vi "Парал-рег.vi"(0 "d 1":bool, 1 "d 2":bool, 2 "d 3":bool, 3 "d 4":bool, 4 "d 5":bool, 7 "Reset":bool, 9 "C":bool) -> (14 "Q 0":bool, 15 "Q 1":bool, 16 "Q 2":bool, 17 "Q 3":bool, 18 "Q 4":bool)   [LabVIEW 2012]
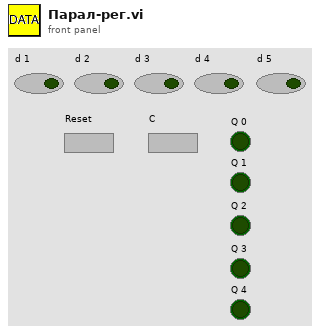
[diagram p1: front panel]
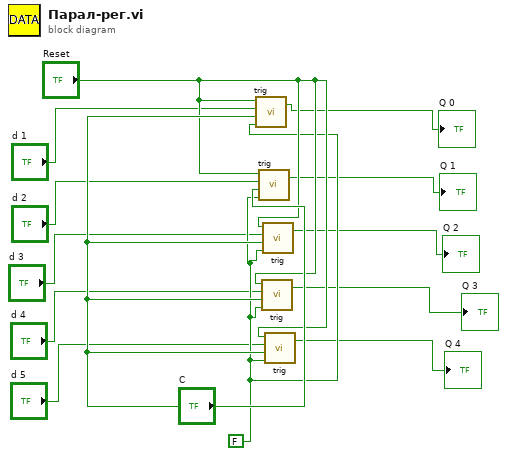
[diagram p0: block diagram]
diagram:
  w11 = FALSE
  n1 = call "trig.vi"("s"=w11, "c"="C", "d"="d 1", "r"="Reset") -> ("q"=→"Q 0":bool)  [unwired: 1 out]
  n2 = call "trig.vi"("s"=w11, "c"="C", "d"="d 2", "r"="Reset") -> ("q"=→"Q 1":bool)  [unwired: 1 out]
  n3 = call "trig.vi"("s"=w11, "c"="C", "d"="d 4", "r"="Reset") -> ("q"=→"Q 3":bool)  [unwired: 1 out]
  n4 = call "trig.vi"("s"=w11, "c"="C", "d"="d 3", "r"="Reset") -> ("q"=→"Q 2":bool)  [unwired: 1 out]
  n5 = call "trig.vi"("s"=w11, "c"="C", "d"="d 5", "r"="Reset") -> ("q"=→"Q 4":bool)  [unwired: 1 out]
